vi "Fault Text.vi"(11 "Boolean":bool) -> (3 "Fault / No Fault":string)   [LabVIEW 2016]
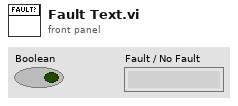
[diagram p1: front panel]
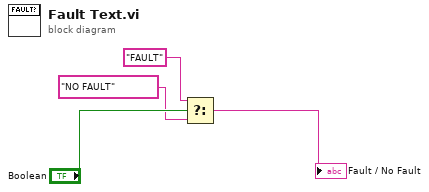
[diagram p0: block diagram]
diagram:
  n1 = Select(t="FAULT", s="Boolean", f="NO FAULT") -> (s? t:f=→"Fault / No Fault":string)
